vi "Path Builder FGV.vi"(0 "State":T1(ring), 1 "Child Folder":string, 5 "Local Path Input":string, 9 "RT Path Input":string) -> (3 "Dup Child Folder Out":string, 4 "Modified Local Out":string, 6 "Root Local Out":string, 8 "Modified RT Out":string, 10 "Root RT Out":string)   [LabVIEW 2023]
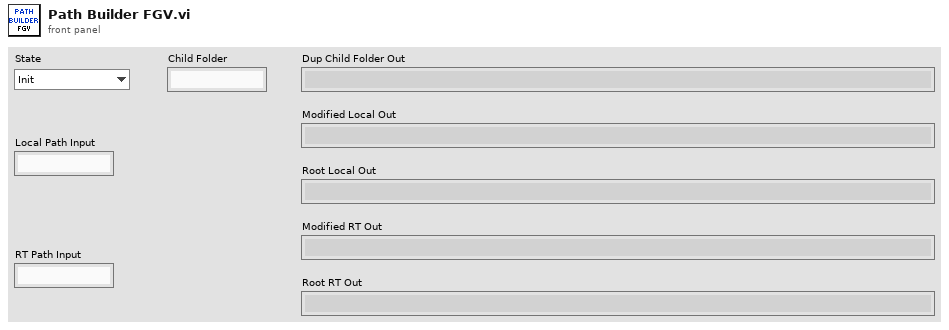
[diagram p1: front panel]
types:
  T1 = enum16{"Init", "Go to Root", "Go Into", "Go Up a Level", "Get Path"}
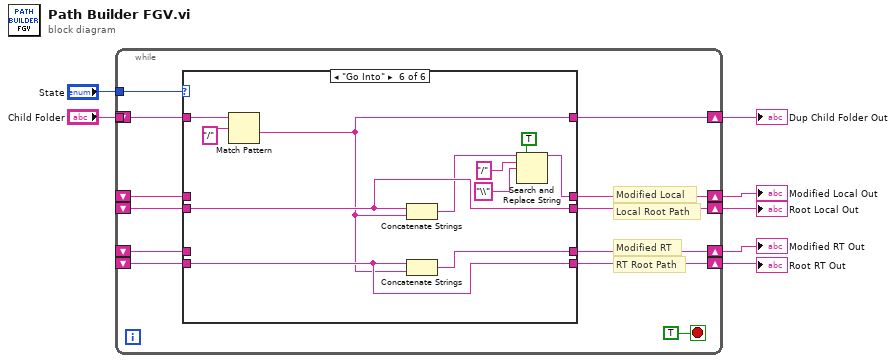
[diagram p0: block diagram]
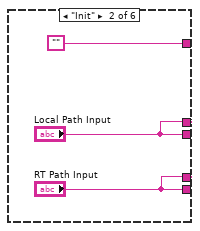
[diagram p3: hidden frame]
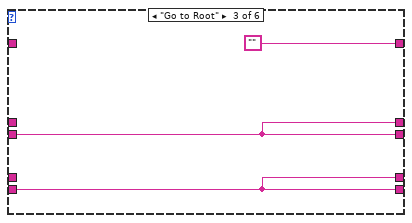
[diagram p4: hidden frame]
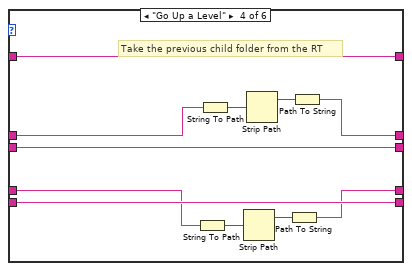
[diagram p5: hidden frame]
diagram:
  n1 = while {
    tunnel: "State" -> [w18]
    shift-right: [w17] -> w3
    shift-left: _ -> [w16]
    shift-right: [w15] -> w2
    shift-left: _ -> [w19]
    shift-right: [w10] -> w5
    shift-left: _ -> [w14]
    shift-right: [w11] -> w4
    shift-left: _ -> [w13]
    shift-right: [w8] -> w1
    shift-left: _ -> [_]
    tunnel: "Child Folder" -> [w9]
    stop <- TRUE stop-if-true
    # "Modified RT"
    # "RT Root Path"
    # "Modified Local"
    # "Local Root Path"
    n2 = case shown="\"Go Into\"" w18 {
      tunnel: w19 -> [w23 _ w30 w40 w45 w56]
      tunnel: [w24 "RT Path Input" w29 w41 w46 w57] -> w17
      tunnel: w16 -> [w24 _ w29 w41 w46 w57]
      tunnel: [w23 "Local Path Input" w30 w40 w45 w56] -> w15
      tunnel: [w22 "Local Path Input" w30 w34 w43 w50] -> w10
      tunnel: w14 -> [w22 _ _ w35 w43 _]
      tunnel: [w21 "RT Path Input" w29 w32 w44 w55] -> w11
      tunnel: w13 -> [w21 _ _ w33 w44 _]
      tunnel: w9 -> [w20 _ _ w31 w42 w49]
      tunnel: [w20 "" "" w31 w42 w47] -> w8
      frame Default {
      }
      frame "Init" {
      }
      frame "Go to Root" {
      }
      frame "Go Up a Level" {
        # "Take the previous child folder from the RT"
        n3 = String To Path(string=w33) -> (path=w36:path)
        n4 = String To Path(string=w35) -> (path=w39:path)
        n5 = Strip Path(path=w36) -> (stripped path=w37:path)  [unwired: 1 out]
        n6 = Strip Path(path=w39) -> (stripped path=w38:path)  [unwired: 1 out]
        n7 = Path To String(path=w37) -> (string=w32:string)
        n8 = Path To String(path=w38) -> (string=w34:string)
      }
      frame "Get Path" {
      }
      frame "Go Into" {
        n9 = Match Pattern(string=w49, regular expression="/") -> (after substring=w47:string)  [unwired: 1 in, 3 out]
        n10 = Concatenate Strings(w56, w47) -> (w51:string)
        n11 = Concatenate Strings(w57, w47) -> (w55:string)
        n12 = Search and Replace String(replace all?=TRUE ("replace all? (F)"), input string=w51, search string="/", replace string="\\" ("replace string (\"\")")) -> (result string=w50:string)  [unwired: 4 in, 3 out]
      }
    }
  }
  "Dup Child Folder Out" <- w1
  "Modified Local Out" <- w5
  "Modified RT Out" <- w4
  "Root RT Out" <- w3
  "Root Local Out" <- w2
